vi "test get all values for sequence.vi"(8 "error in":errorcluster, 11 "cycle results cluster IN":T1) -> (0 "Sequence Results":dbl[][](array[numeric]), 3 "cycle results cluster out":T1)   [LabVIEW 2016]
doc: "Takes a sample type and sorts by sequence"
uses:
  controls/cycle results control.ctl
  <vilib>/Analysis/baseanly.llb/Mean (DBL).vi
  <vilib>/Analysis/NI_AALBase.lvlib
panel:
  out "Array 8":dbl[][](array[numeric])
  out "Array 7":dbl[](array[numeric])
  out "Array 6":dbl[][](array[numeric])
  out "Array 5":dbl[][](array[numeric])
  out "Array 4":dbl[][](array[numeric])
  out "Array 3":dbl[][](array[numeric])
  out "appended array":dbl[][](array[numeric])
  out "Array 2":dbl[](array[numeric])
  out "Array":dbl[][][](array[numeric])
  in  "cycle results cluster test":T1 {"cycle results dbl" format="%#_6e"}
  out "error out":errorcluster
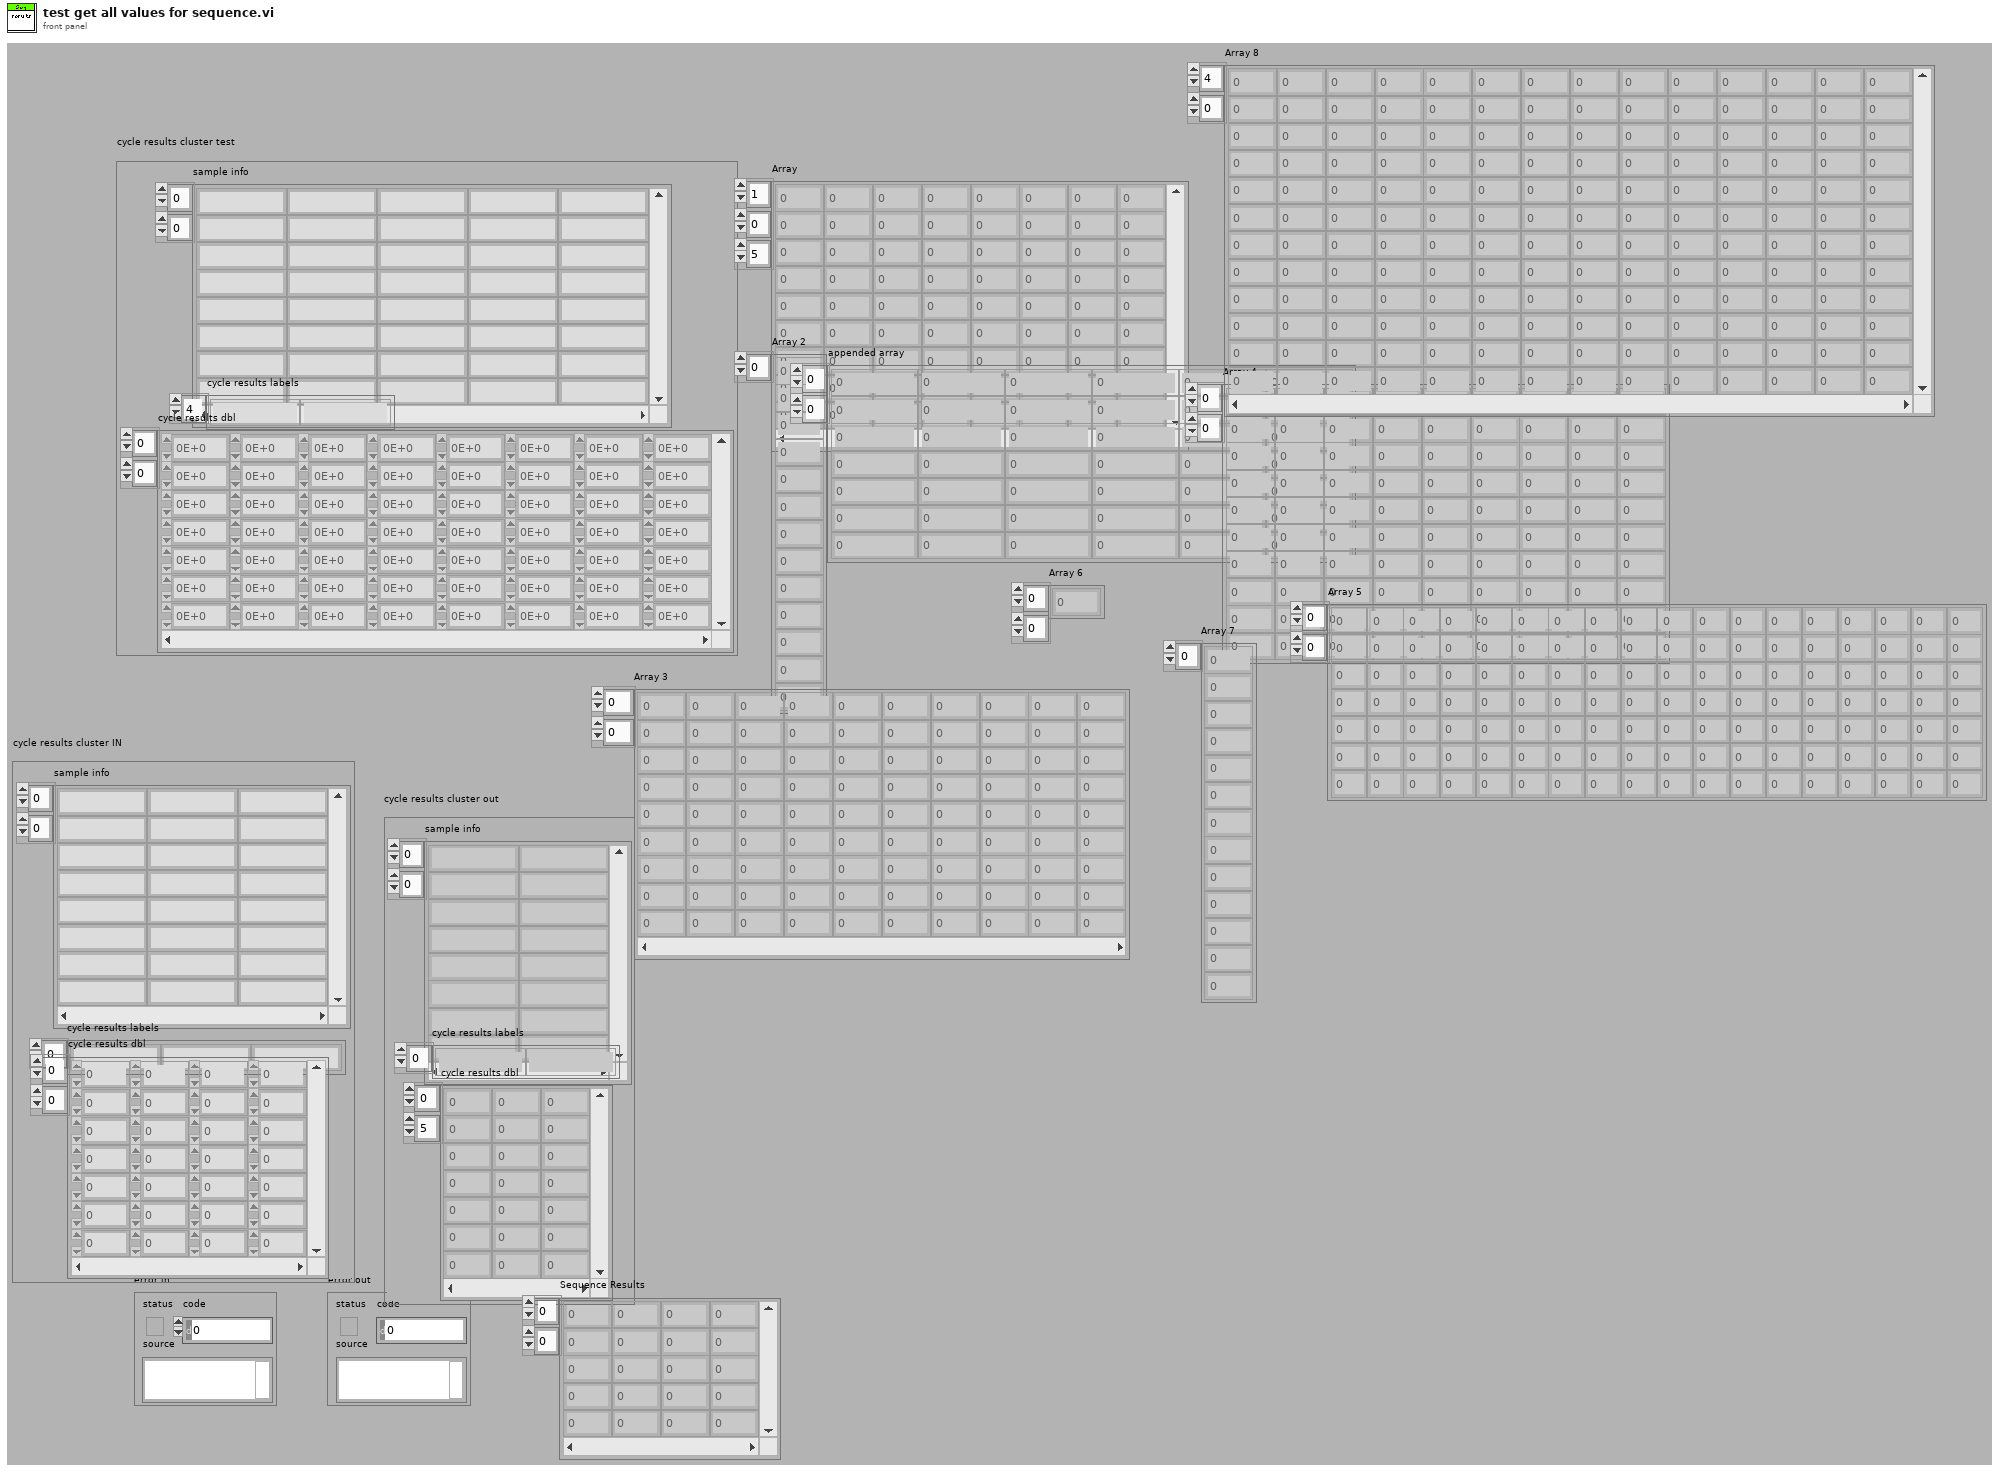
[diagram p1: front panel]
types:
  T1 = typedef "cycle results control.ctl" = cluster{"sample info":string[][], "cycle results labels":string[], "cycle results dbl":dbl[][]}
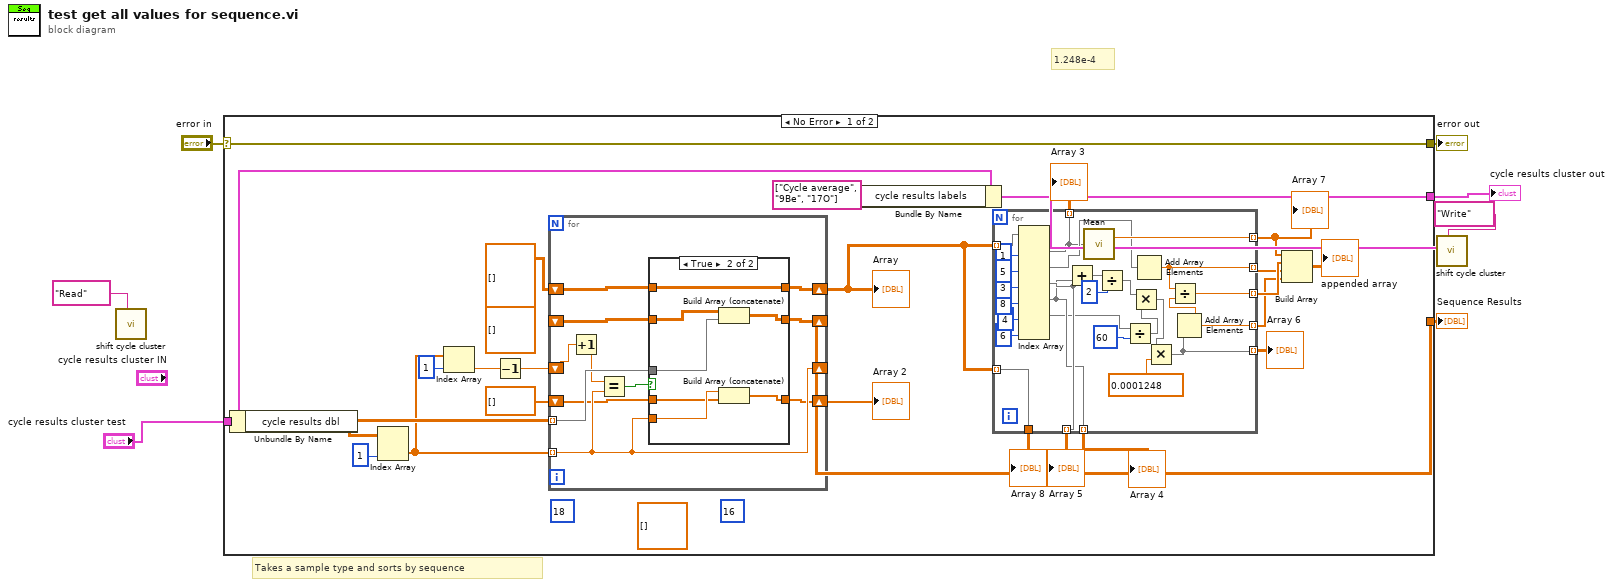
[diagram p0: block diagram]
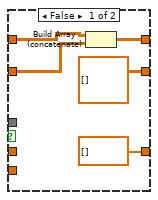
[diagram p2: hidden frame]
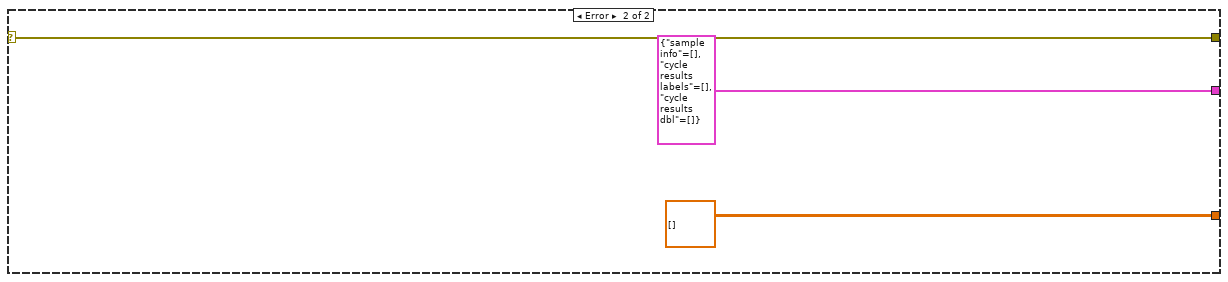
[diagram p3: hidden frame]
diagram:
  # "1.248e-4"
  # "Takes a sample type and sorts by sequence"
  n1 = call "shift cycle cluster.vi"("read write shift"="Read") -> ()  [unwired: 9 in, 2 out]
  n2 = case shown="No Error" "error in" {
    selector: "error in" -> [w30 w82]
    tunnel: "cycle results cluster test" -> [w29 _]
    tunnel: [w21 dbl[][] []] -> w2
    tunnel: [w27 T1 {"sample info"=[], "cycle results labels"=[], "cycle results dbl"=[]} ("cycle results cluster IN")] -> w3
    tunnel: [w30 w82] -> w6
    frame No Error {
      (unwired) dbl[][] []
      (unwired) 18 ("index (col)")
      (unwired) 16 ("index (col)")
      (unwired) dbl[][] []
      n3 = Unbundle By Name(w29) -> ("cycle results dbl"=w26:dbl[][])
      n4 = Index Array(array=w26, index (col)=1 ("disabled index (col)")) -> (element=w23:dbl[])  [unwired: 1 in]
      n5 = Index Array(array=w23, index=1) -> (element=w25:dbl)
      n6 = Decrement(x=w25) -> (x-1=w24:dbl)
      n7 = for {
        tunnel: w26 -> [w67] mode=indexing
        tunnel: w23 -> [w66] mode=indexing
        shift-right: [w66] -> _
        shift-left: w24 -> [w59]
        shift-right: [w65] -> w20
        shift-left: dbl[] [] -> [w64]
        shift-right: [w63] -> w21
        shift-left: _ -> [w62]
        shift-right: [w61] -> w9
        shift-left: dbl[][][] [] -> [w60]
        n8 = Increment(x=w59) -> (x+1=w58:dbl)
        n9 = Equal?(x=w58, y=w66) -> (x = y?=w68:bool)
        n10 = case shown="True" w68 {
          tunnel: w66 -> [_ w80]
          tunnel: w67 -> [_ w75]
          tunnel: [dbl[] [] w79] -> w65
          tunnel: w64 -> [_ w78]
          tunnel: [dbl[][] [] w77] -> w63
          tunnel: w62 -> [w69 w74]
          tunnel: [w71 w76] -> w61
          tunnel: w60 -> [w70 w76]
          frame False {
            n11 = Build Array (concatenate)(w70, w69) -> (w71:dbl[][][])
          }
          frame True {
            n12 = Build Array (concatenate)(w74, w75) -> (w77:dbl[][])
            n13 = Build Array (concatenate)(w80, w78) -> (w79:dbl[])
          }
        }
      }
      "Array" <- w9
      "Array 2" <- w20
      n14 = Bundle By Name(cluster=w29, "cycle results labels"=string[] ["Cycle average", "9Be", "17O"]) -> (w27:T1)
      n15 = for {
        tunnel: w9 -> [w57] mode=indexing
        tunnel: [w51] -> w17 mode=indexing
        tunnel: [w46] -> w18 mode=indexing
        tunnel: [w34] -> w15 mode=indexing
        tunnel: [w45] -> w13 mode=indexing
        tunnel: [w44] -> w14 mode=indexing
        tunnel: [w43] -> w11 mode=indexing
        tunnel: [w42] -> w12 mode=indexing
        tunnel: [w36] -> w10 mode=indexing
        tunnel: w9 -> [w33] mode=indexing
        tunnel: [w33] -> w8
        n16 = Index Array(array=w57, index (col) #1=1 ("disabled index (col)"), index (col) #2=5 ("disabled index (col)"), index (col) #3=3 ("index (col)"), index (col) #4=8 ("index (col)"), index (col) #5=4 ("index (col)"), index (col) #6=6 ("index (col)")) -> (element #1=w34:dbl[], element #2=w35:dbl[], element #3=w43:dbl[], element #4=w42:dbl[], element #5=w39:dbl[])  [unwired: 6 in, 1 out]
        n17 = Add(x=w43, y=w42) -> (x+y=w40:dbl[])
        n18 = call-poly <vilib>:"Mean.vi"("X"=w34) -> ("mean"=w51:dbl)  [unwired: 1 out]
        n19 = Divide(x=w40, y=2 ("String")) -> (x/y=w49:dbl[])
        n20 = Divide(x=w39, y=60 ("String")) -> (x/y=w47:dbl[])
        n21 = Multiply(x=w49, y=w47) -> (x*y=w38:dbl[])
        n22 = Add Array Elements(numeric array=w35) -> (sum=w44:dbl)
        n23 = Multiply(x=w38, y=0.0001248 ("String")) -> (x*y=w36:dbl[])
        n24 = Add Array Elements(numeric array=w36) -> (sum=w45:dbl)
        n25 = Divide(x=w44, y=w45) -> (x/y=w46:dbl)
      }
      "Array 3" <- w15
      "Array 4" <- w12
      "Array 5" <- w11
      "Array 6" <- w10
      "Array 7" <- w17
      "Array 8" <- w8
      n26 = Build Array(w17, w18, w14, w13) -> (→"appended array":dbl[][])
    }
    frame Error {
    }
  }
  "error out" <- w6
  "cycle results cluster out" <- w3
  "Sequence Results" <- w2
  n27 = call "shift cycle cluster.vi"("read write shift"="Write", "cycle results cluster In"=w3) -> ()  [unwired: 8 in, 2 out]
